vi "Init.vi"(6 "Array":T9[](array[typedef]) {"MinWidth" min=2 step=1; "AutoSizeMode" items=["None"=1, "ColumnHeader"=2, "AllCellsExceptHeader"=4, "AllCells"=6, "DisplayedCellsExceptHeader"=8, "DisplayedCells"=10, "Fill"=16]; "FillWeight" min=1 max=100}, 8 "error in":errorcluster, 9 "object refs":T8, 10 "References in":T1, 11 "Data Grid in":refnum<class "Data Grid.lvclass">) -> (0 "error out":errorcluster, 2 "Registered Events":refnum<event-registration>, 3 "Data Grid out":refnum<class "Data Grid.lvclass">)   [LabVIEW 2013, in "Table Manager.lvlib" / "Data Grid.lvclass"]
uses:
  Data Grid.lvclass
  <vilib>/NI/Tag Bus/tag/tag descriptor.lvclass
  <vilib>/NI/Tag Bus Module Framework/channel/TBM channel.lvclass
  <vilib>/NI/DCAF/Tag Editor Core/control module/editor node/dialog output action.ctl
  <vilib>/NI/DCAF/Tag Editor Core/control module/editor node/control module editor.lvclass
  <vilib>/NI/DCAF/Tag Editor Core/control module/editor node/channel action event.ctl
  <vilib>/DataGrid for LabVIEW/source/Events/Abstract EVENT/Abstract EVENT.lvclass
  <vilib>/NI/Configuration Framework/Node/StopEvent.ctl
  <vilib>/NI/Configuration Framework/Node/NISE_CEF_Node.lvclass
  <vilib>/NI/Configuration Framework/Node/RefreshUIEvent.ctl
  <vilib>/NI/Configuration Framework/Node/CacheState.ctl
  <vilib>/NI/Configuration Framework/Node/NodeRef.ctl
  <vilib>/NI/Configuration Framework/Node/NodeChangeEvent.ctl
  <vilib>/NI/Configuration Framework/Controls/EventCluster.ctl
  <vilib>/NI/Configuration Framework/NISE_CEF_TreeControl.lvlib
  <vilib>/NI/Configuration Framework/Node/UserEventRef.ctl
  Internal Reg Events.ctl
  Table Manager.lvlib
  Line/Line.lvclass
  String Column/String Column.lvclass
  Mapping Column/Mapping Column.lvclass
  DataGridEnum Column/DataGridEnum Column.lvclass
  <vilib>/DataGrid for LabVIEW/source/GridColumn/ColumnType.ctl
  <vilib>/DataGrid for LabVIEW/source/GridColumn/GridColumn.lvclass
  <vilib>/DataGrid for LabVIEW/source/GridColumn/ColumnDefinition.ctl
  Program Files (x86)/National Instruments/LabVIEW 2013/examples/DataGrid for LabVIEW/DataGrid.lvlib
  <vilib>/NI/Tag Bus/tag/Data Type.ctl
  Column/Column Descriptor.ctl
  Column/Column.lvclass
  <vilib>/NI/DCAF/Tag Editor Core/Configuration Editor/Classes/Engine Parent/Engine Parent Editor Node.lvclass
  Table Manager/object ref.ctl
  Table Manager/Table Manager.lvclass
  <vilib>/NI/Tools/Keyed Array/KeyedArray.ctl
  <vilib>/NI/Tools/Keyed Array/Tools_KeyedArray.lvlib
  <vilib>/NI/AMC/Message.ctl
  <vilib>/NI/AMC/AMC.lvlib
  <vilib>/NI/AMC/Message Queue.ctl
  Table Manager/references.ctl
  Column/Column Type.ctl
  <vilib>/NI/DCAF/Tag Editor Core/Configuration Editor/Classes/Module editor node/module editor node.lvclass
  Table Manager/Call Back Ref Type Def.ctl
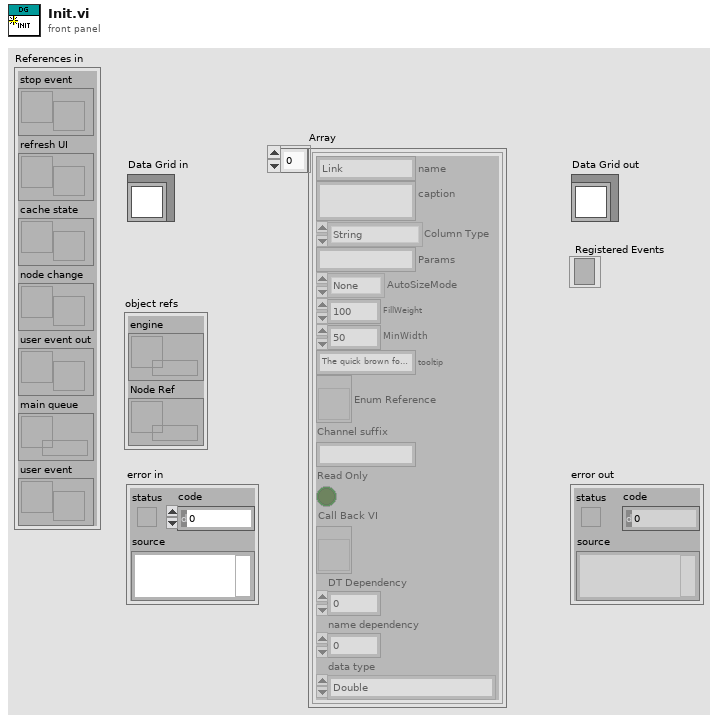
[diagram p1: front panel]
types:
  T1 = typedef "Table Manager.lvlib/Table Manager.lvclass/references.ctl" = cluster{"stop event":T2, "refresh UI":T3, "cache state":T4, "node change":T5, "user event out":refnum<user-event>, "main queue":T6, "user event":T7}
  T2 = typedef "NISE_CEF_Node.lvclass/StopEvent.ctl" = refnum<user-event>
  T3 = typedef "NISE_CEF_Node.lvclass/RefreshUIEvent.ctl" = refnum<user-event>
  T4 = typedef "NISE_CEF_Node.lvclass/CacheState.ctl" = refnum<user-event>
  T5 = typedef "NISE_CEF_Node.lvclass/NodeChangeEvent.ctl" = refnum<user-event>
  T6 = typedef "AMC.lvlib/Message Queue.ctl" = refnum<queue>
  T7 = typedef "NISE_CEF_Node.lvclass/UserEventRef.ctl" = refnum<user-event>
  T8 = typedef "Table Manager.lvlib/Table Manager.lvclass/object ref.ctl" = cluster{"engine":refnum<data-value>, "Node Ref":refnum<data-value>}
  T9 = typedef "Table Manager.lvlib/Column.lvclass/Column Descriptor.ctl" = cluster{"name":string, "caption":string, "Column Type":T10, "Params":string, "AutoSizeMode":i32, "FillWeight":sgl, "MinWidth":u32, "tooltip":string, "Enum Reference":refnum<vi>, "Channel suffix":string, "Read Only":bool, "Call Back VI":T11, "DT Dependency":i32, "name dependency":i32, "data type":T12}
  T10 = typedef "Table Manager.lvlib/Column.lvclass/Column Type.ctl" = enum16{"String", "Mapping", "Channel Name", "Tag", "Enum", "Data Type", "Numeric"}
  T11 = typedef "Table Manager.lvlib/Table Manager.lvclass/Call Back Ref Type Def.ctl" = refnum<vi>
  T12 = typedef "tag bus.lvlib/tag descriptor.lvclass/Data Type.ctl" = enum16{"Double", "Single", "I64", "I32", "I16", "I8", "U64", "U32", "U16", "U8", "Boolean", "String", "Array of Double", "Array of Single", "Array of I64", "Array of I32", "Array of I16", "Array of I8", "Array of U64", "Array of U32", "Array of U16", "Array of U8", "Array of Boolean", "Array of String"}
  T13 = typedef "Table Manager.lvlib/Internal Reg Events.ctl" = cluster{"Data Grid":refnum<event-registration>, "Node Events":refnum<event-registration>}
  T14 = typedef "control module editor.lvclass/channel action event.ctl" = cluster{"action":T15, "channel":refnum<class "TBM channel.lvclass">, "selected tag":refnum<class "tag descriptor.lvclass">}
  T15 = typedef "control module editor.lvclass/dialog output action.ctl" = enum16{"Tag Created", "Tag Selected", "Set Default", "disconnect"}
  T16 = typedef "DataGrid.lvlib/GridColumn.lvclass/ColumnDefinition.ctl" = cluster{"name":string, "caption":string, "datatype":T17, "Params":string, "AutoSizeMode":i32, "FillWeight":sgl, "MinWidth":u32, "tooltip":string}
  T17 = typedef "DataGrid.lvlib/GridColumn.lvclass/ColumnType.ctl" = enum16{"string", "image", "check", "numeric", "timestamp", "button", "combo", "link"}
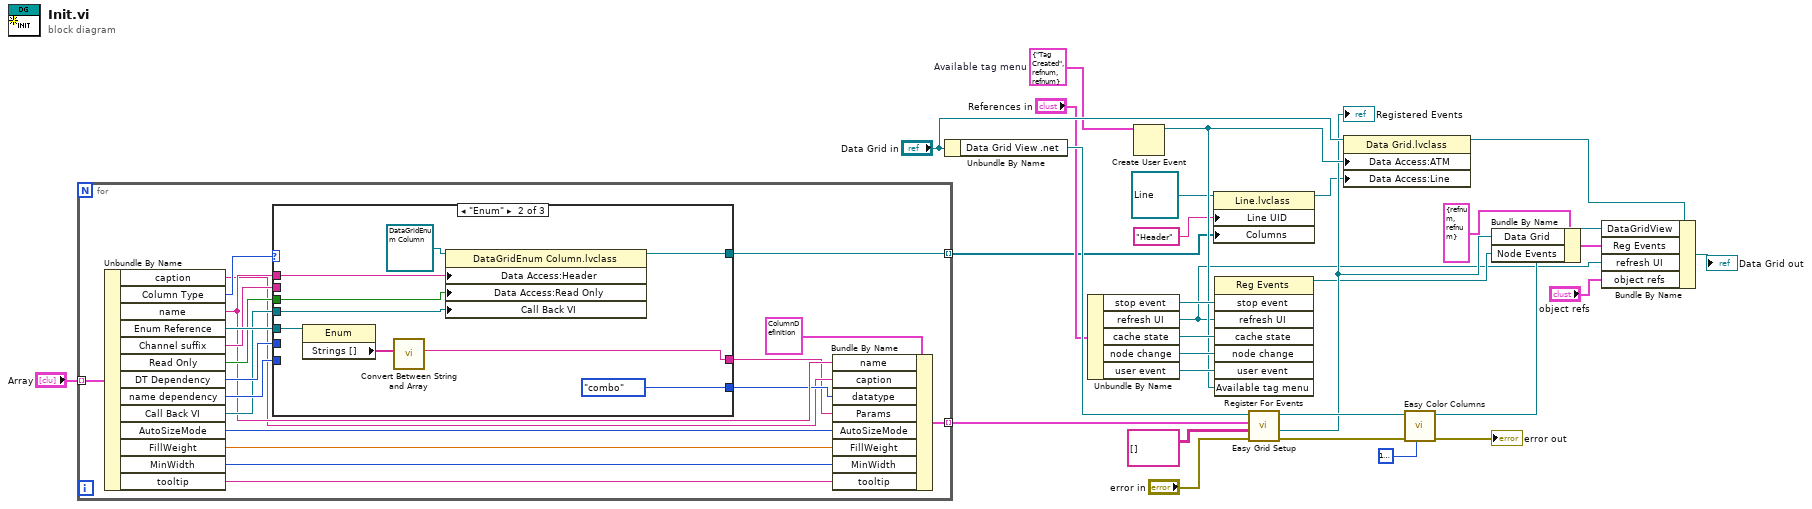
[diagram p0: block diagram]
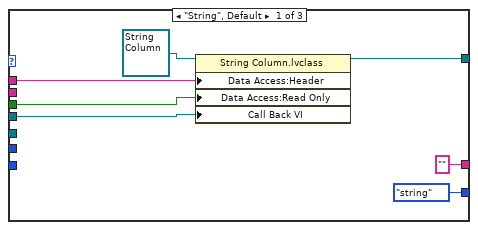
[diagram p2: hidden frame]
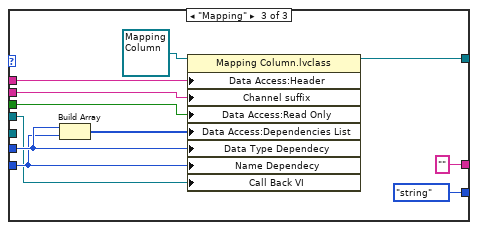
[diagram p3: hidden frame]
diagram:
  w19 = T14 {"action"=enum."Tag Created", "channel"=refnum, "selected tag"=refnum}  # Available tag menu
  n1 = for {
    tunnel: "Array" -> [w49] mode=indexing
    tunnel: [w47] -> w2 mode=indexing
    tunnel: [w39] -> w3 mode=indexing
    n2 = Unbundle By Name(w49) -> ("caption"=w32:string, "Column Type"=w48:T10, "name"=w38:string, "Enum Reference"=w46:refnum<vi>, "Channel suffix"=w45:string, "Read Only"=w44:bool, "DT Dependency"=w43:i32, "name dependency"=w42:i32, "Call Back VI"=w41:T11, "AutoSizeMode"=w34:i32, "FillWeight"=w35:sgl, "MinWidth"=w36:u32, "tooltip"=w37:string)
    n3 = case shown="\"Enum\"" w48 {
      tunnel: [w54 w65 w75] -> w47
      tunnel: w38 -> [w55 w64 w74]
      tunnel: w46 -> [_ w59 _]
      tunnel: w45 -> [_ _ w73]
      tunnel: w44 -> [w53 w63 w72]
      tunnel: w43 -> [_ _ w70]
      tunnel: w42 -> [_ _ w69]
      tunnel: w41 -> [w52 w62 w68]
      tunnel: [ColumnType."string" ("datatype") ColumnType."combo" ("datatype") ColumnType."string" ("datatype")] -> w33
      tunnel: ["" ("Params") w57 "" ("Params")] -> w31
      frame "String", Default {
        n4 = property class="String Column.lvclass"(reference=refnum<class "String Column.lvclass"> refnum ("Table Manager.lvlib:String Column.lvclass"), "Data Access:Header"=w55, "Data Access:Read Only"=w53, "Call Back VI"=w52) -> (reference out=w54:refnum<class "String Column.lvclass">)  [unwired: 1 in, 1 out]
      }
      frame "Enum" {
        n5 = property class="Enum"(reference=w59) -> ("Strings []"=w58:string[])  [unwired: 1 in, 2 out]
        n6 = call <vilib>:"Convert Between String and Array.vi"("String Array"=w58) -> ("String"=w57:string)  [unwired: 9 in, 1 out]
        n7 = property class="DataGridEnum Column.lvclass"(reference=refnum<class "DataGridEnum Column.lvclass"> refnum ("Table Manager.lvlib:DataGridEnum Column.lvclass"), "Data Access:Header"=w64, "Data Access:Read Only"=w63, "Call Back VI"=w62) -> (reference out=w65:refnum<class "DataGridEnum Column.lvclass">)  [unwired: 1 in, 1 out]
      }
      frame "Mapping" {
        n8 = Build Array(w70, w69) -> (w71:i32[])
        n9 = property class="Mapping Column.lvclass"(reference=refnum<class "Mapping Column.lvclass"> refnum ("Table Manager.lvlib:Tag Channel Column.lvclass"), "Data Access:Header"=w74, "Channel suffix"=w73, "Data Access:Read Only"=w72, "Data Access:Dependencies List"=w71, "Data Type Dependecy"=w70, "Name Dependecy"=w69, "Call Back VI"=w68) -> (reference out=w75:refnum<class "Mapping Column.lvclass">)  [unwired: 1 in, 1 out]
      }
    }
    n10 = Bundle By Name(cluster=T16 {"name"="Selector Name", "caption"="", "datatype"=enum."string", "Params"="", "AutoSizeMode"=16, "FillWeight"=100.0, "MinWidth"=50, "tooltip"="Name for the selector"}, "name"=w38, "caption"=w32, "datatype"=w33, "Params"=w31, "AutoSizeMode"=w34, "FillWeight"=w35, "MinWidth"=w36, "tooltip"=w37) -> (w39:T16)
  }
  n11 = Unbundle By Name("Data Grid in") -> ("Data Grid View .net"=w22:refnum<k24>)
  n12 = Unbundle By Name("References in") -> ("stop event"=w17:T2, "refresh UI"=w8:T3, "cache state"=w16:T4, "node change"=w15:T5, "user event"=w14:T7)
  n13 = Create User Event(user event datatype=w19) -> (user event=w13:refnum<user-event>)  [unwired: 1 in, 1 out]
  n14 = property class="Line.lvclass"(reference=refnum<class "Line.lvclass"> refnum ("Table Manager.lvlib:Line.lvclass"), "Line UID"="Header", "Columns"=w2) -> (reference out=w1:refnum<class "Line.lvclass">)  [unwired: 1 in, 1 out]
  n15 = register-events(w17, w8, w16, w15, w14, w13) -> (reference out=w10:refnum<event-registration>)  [unwired: 2 in, 1 out]
  n16 = call <vilib>:"Easy Grid Setup.vi"("error in"="error in", "DataSource Data"=string[][] [], "ColumnSetup"=w3, "DataGridView"=w22) -> ("error out"=w30:errorcluster, "registeredEvents"=w11:refnum<event-registration>, "DataGrid out"=w29:refnum<class "DataGridView.lvclass">)  [unwired: 4 in, 1 out]
  "Registered Events" <- w11
  n17 = property class="Data Grid.lvclass"(reference="Data Grid in", "Data Access:ATM"=w13, "Data Access:Line"=w1) -> (reference out=w20:refnum<class "Data Grid.lvclass">)  [unwired: 1 in, 1 out]
  n18 = call <vilib>:"Easy Color Columns.vi"("BGK Color"=u32 16777224, "error in (no error)"=w30, "DataGridView in"=w29) -> ("error out"=→"error out":errorcluster, "DataGridView out"=w27:refnum<class "DataGridView.lvclass">)  [unwired: 7 in]
  n19 = Bundle By Name(cluster=T13 {"Data Grid"=refnum, "Node Events"=refnum} ("Reg Events"), "Data Grid"=w11, "Node Events"=w10) -> (w9:T13)
  n20 = Bundle By Name(cluster=w20, "DataGridView"=w27, "Reg Events"=w9, "refresh UI"=w8, "object refs"="object refs") -> (→"Data Grid out":refnum<class "Data Grid.lvclass">)
